vi "Copy gplugin file.vi"(0 "Config":T1, 5 "Plugin Path":path, 11 "error in (no error)":errorcluster) -> (4 "G PLugin File Path":path, 15 "error out":errorcluster)   [LabVIEW 2021, in "G Plugin Editor.lvlib"]
uses:
  G Plugin Editor.lvlib
  controls/Data Holder.ctl
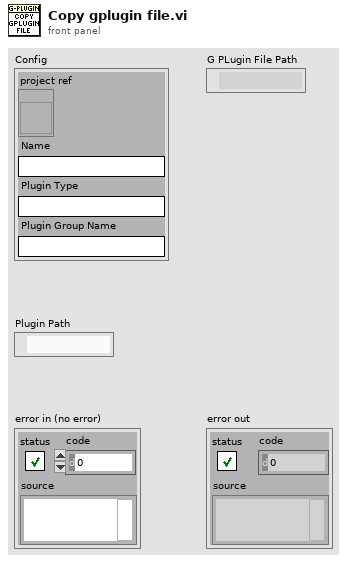
[diagram p1: front panel]
types:
  T1 = typedef "G Plugin Editor.lvlib/Data Holder.ctl" = cluster{"project ref":refnum<vi>, "Name":string, "Plugin Type":string, "Plugin Group Name":string}
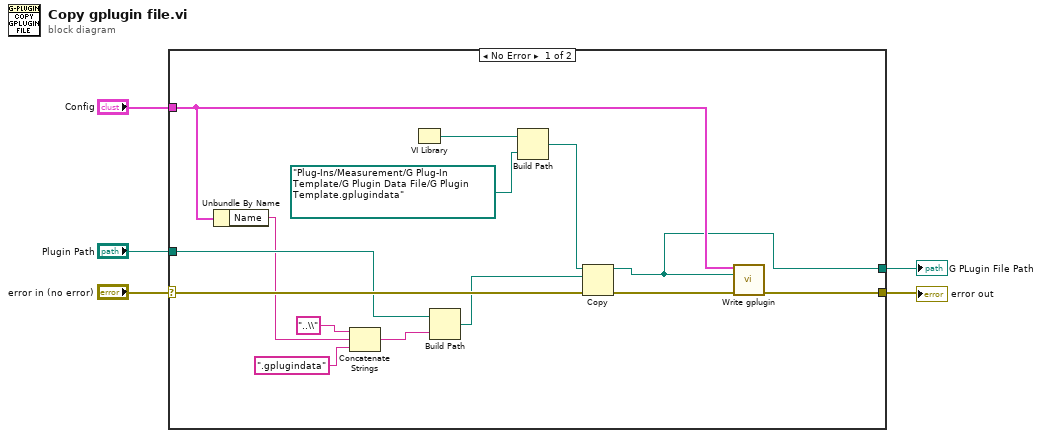
[diagram p0: block diagram]
diagram:
  n1 = case shown="No Error" "error in (no error)" {
    selector: "error in (no error)" -> [w19 w20]
    tunnel: [w12 w20] -> w5
    tunnel: [w10 _] -> w3
    tunnel: "Plugin Path" -> [w15 _]
    tunnel: "Config" -> [w13 _]
    frame No Error {
      n2 = Unbundle By Name(w13) -> ("Name"=w14:string)
      n3 = Concatenate Strings("..\\" ("string"), w14, ".gplugindata" ("string")) -> (w17:string)
      n4 = VI Library() -> (path=w8:path)
      n5 = Build Path(base path=w15, name or relative path=w17) -> (appended path=w18:path)
      n6 = Build Path(base path=w8, name or relative path=path "Plug-Ins/Measurement/G Plug-In Template/G Plugin Data File/G Plugin Template.gplugindata") -> (appended path=w6:path)
      n7 = Copy(8:w19, 10:w18, 11:w6) -> (0:w11:errorcluster, 3:w10:path)  [unwired: 2 in, 1 out]
      n8 = call "Write gplugin.vi"("Config"=w13, "Path"=w10, "error in (no error)"=w11) -> ("error out"=w12:errorcluster)  [unwired: 12 in]
    }
    frame Error {
    }
  }
  "error out" <- w5
  "G PLugin File Path" <- w3
